vi "LCAIO Set Input Sw Scaling On.vi"(7 "Scaling On":bool, 8 "error in (no error)":errorcluster caption="Fehler (Eingang, kein Fehler)", 11 "Input Channel Handle":i64) -> (0 "error out":errorcluster caption="Fehler (Ausgang)")   [LabVIEW 2021, in "labbCAN_AnalogIO_API.lvlib"]
doc: "LCAIO_Func long LCAIO_CALL LCAIO_SetInputSwScalingOn(dev_hdl InChanHdl,\n unsigned char ScalingOn);"
uses:
  labbCAN_AnalogIO_API.lvlib
  labbCAN_AnalogIO_API.dll
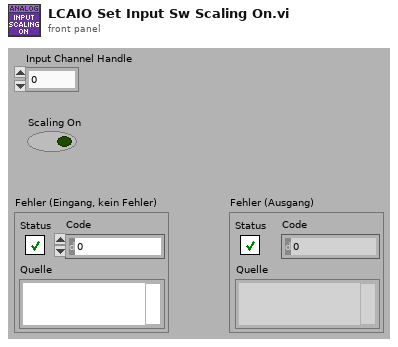
[diagram p1: front panel]
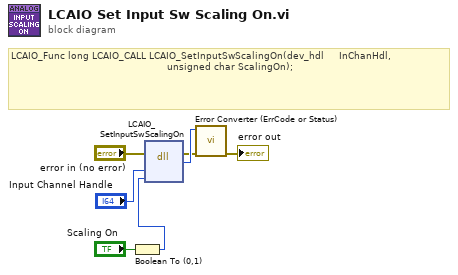
[diagram p0: block diagram]
diagram:
  # "LCAIO_Func long LCAIO_CALL LCAIO_SetInputSwScalingOn(dev_hdl     InChanHdl,\n                                                    unsigned char ScalingOn);"
  n1 = Boolean To (0,1)(Boolean="Scaling On") -> (0, 1=w1:i16)
  n2 = dll-call lib="C:/Users/olaja/AppData/Local/CETONI_SDK/labbCAN_AnalogIO_API.*" fn="LCAIO_SetInputSwScalingOn"(error in="error in (no error)", "Input Channel Handle"="Input Channel Handle", "Scaling On"=w1) -> (error out=w4:errorcluster, "Rückgabetyp"=w5:i32)  [unwired: 4 in, 1 out]
  n3 = call "Error Converter (ErrCode or Status).vi"("error in (no error)"=w4, "error code"=w5) -> ("error out"=→"error out":errorcluster)  [unwired: 9 in]
